vi "GetFileSpace.vi"() -> ()   [LabVIEW 2010]
uses:
  <vilib>/addons/h5labview2/dataset/H5D.lvlib
  <vilib>/addons/h5labview2/dataset/H5Dwrite.llb/H5Dwrite.xnode
  <vilib>/addons/h5labview2/space/H5S.lvlib
  <vilib>/addons/h5labview2/base/H5Equery.vi
  <vilib>/addons/h5labview2/base/lib_path.vi
  <vilib>/addons/h5labview2/base/hid_t.ctl
  fpga-bitfile-ref.ctl
panel:
  in  "Exp_params":T3={"filename"="201612011532", "ExpFilePath"=path "\\\\10.0.0.7\\takada2/DATA/HBT6/data/Test/201612011532.h5", "File Ref list"=[16777216, 33554432], "sweep_dim"=[4, 2], "sweep_list"=[], "readout_list"=["ADC0", "ADC1"], "Sweep instrument bools"=[[0, 0], [0, 0], [0, 0], [0, 0], [0, 0], [0, 0], [0, 0], [0, 0], [0, 0], [0, 0], [0, 0], [0, 0], [0, 0], [0, 0], [0, 0], [0, 0], [0, 0], [0, 0], [0, 0], [0, 0], [0, 0], [0, 0], [0, 0], [0, 0], [0, 0], [0, 0], [0, 0], [0, 0], [0, 0], [0, 0], [0, 0]], "Read out instrument bools"=[[1, 0]], "Experimental bool list"=[FALSE, TRUE], "Initial move"=[{"Name"="None", "kind"=100, "Value"=0.0}], "FPGA Ref"=refnum, "Inst_parameters"={"ConfigFilePath"=path "\\\\10.0.0.7\\takada2/DATA/HBT6/data/Configs/HBT6_ramp_1.h5", "Inst_list"=["ADC", "AWG", "Freq", "Power", "sus", "rus", "rls", "sls", "suq", "suu", "sur", "suc", "sul", "ruq", "ruu", "rur", "ruc", "rul", "rlq", "rlu", "rlr", "rlc", "rll", "slq", "slu", "slr", "slc", "sll", "tu", "t", "tl", "fast_sequence"], "fast_mode"=[1, 1], "Wait_times"=[1, 1, 1, 1], "Inst_array"=[{"Kind"=0, "Strings"=["ADC", "", "V", "ADC0;ADC1", "V;V", "1.0;1.0"], "uint64s"=[10, 2, 250000, 0, 100, 10106, 1000000, 1, 0, 1], "Doubles"=[1.0], "DAQmx take out list"=[]}, {"Kind"=7, "Strings"=["AWG", "10.0.0.4", "", "C:\\Documents and Settings\\Bauerle\\Mes documents\\Bautze\\FPGA-clean_works_1.13.6_batchtest\\Python\\AWG", "dummy", "SAWnstrig_v4.py"], "uint64s"=[2, 0, 0, 3, 0, 0, 0, 0, 0, 0, 0, 0, 0, 0], "Doubles"=[1200000000.0, 1.0, 0.0, 1.0, 0.0, 1.0, 0.0, 1.0, 0.0, 1.0, 0.0, 1.0, 0.0], "DAQmx take out list"=[]}, {"Kind"=6, "Strings"=["Freq", "0:19", "GHz"], "uint64s"=[1, 0, 0, 0, 2, 0, 0, 0], "Doubles"=[2.0, -30.0, 200.0, 100.0, 0.0, 6.000999927520752, 9.000000318337698e-06, 30.0, -145.0], "DAQmx take out list"=[]}, {"Kind"=6, "Strings"=["Power", "0:19", "GHz"], "uint64s"=[1, 0, 1, 0, 2, 0, 0, 0], "Doubles"=[2.0, -30.0, 200.0, 100.0, 0.0, 6.000999927520752, 9.000000318337698e-06, 30.0, -145.0], "DAQmx take out list"=[]}, {"Kind"=4, "Strings"=["sus", "10.0.0.2", "mV"], "uint64s"=[0, 1], "Doubles"=[1.0, -1.0, 1.0, -1.0, 1.0], "DAQmx take out list"=[]}, {"Kind"=4, "Strings"=["rus", "10.0.0.2", "mV"], "uint64s"=[0, 2], "Doubles"=[1.0, -1.0, 1.0, -1.0, 1.0], "DAQmx take out list"=[]}, {"Kind"=4, "Strings"=["rls", "10.0.0.2", "mV"], "uint64s"=[0, 3], "Doubles"=[1.0, -1.0, 1.0, -1.0, 1.0], "DAQmx take out list"=[]}, {"Kind"=4, "Strings"=["sls", "10.0.0.2", "mV"], "uint64s"=[0, 4], "Doubles"=[1.0, -1.0, 1.0, -1.0, 1.0], "DAQmx take out list"=[]}, {"Kind"=4, "Strings"=["suq", "10.0.0.2", "V"], "uint64s"=[0, 5], "Doubles"=[0.30000001192092896, -2.0, 1.0, -1.0, 1.0], "DAQmx take out list"=[]}, {"Kind"=4, "Strings"=["suu", "10.0.0.2", "V"], "uint64s"=[0, 6], "Doubles"=[0.30000001192092896, -2.0, 1.0, -1.0, 1.0], "DAQmx take out list"=[]}, {"Kind"=4, "Strings"=["sur", "10.0.0.2", "V"], "uint64s"=[0, 7], "Doubles"=[0.30000001192092896, -2.0, 1.0, -1.0, 1.0], "DAQmx take out list"=[]}, {"Kind"=4, "Strings"=["suc", "10.0.0.2", "V"], "uint64s"=[1, 0], "Doubles"=[0.30000001192092896, -2.0, 1.0, -1.0, 1.0], "DAQmx take out list"=[]}, {"Kind"=4, "Strings"=["sul", "10.0.0.2", "V"], "uint64s"=[1, 1], "Doubles"=[0.30000001192092896, -2.0, 1.0, -1.0, 1.0], "DAQmx take out list"=[]}, {"Kind"=4, "Strings"=["ruq", "10.0.0.2", "V"], "uint64s"=[1, 2], "Doubles"=[0.30000001192092896, -2.0, 1.0, -1.0, 1.0], "DAQmx take out list"=[]}, {"Kind"=4, "Strings"=["ruu", "10.0.0.2", "V"], "uint64s"=[1, 3], "Doubles"=[0.30000001192092896, -2.0, 1.0, -1.0, 1.0], "DAQmx take out list"=[]}, {"Kind"=4, "Strings"=["rur", "10.0.0.2", "V"], "uint64s"=[1, 5], "Doubles"=[0.30000001192092896, -2.0, 1.0, -1.0, 1.0], "DAQmx take out list"=[]}, {"Kind"=4, "Strings"=["ruc", "10.0.0.2", "V"], "uint64s"=[1, 6], "Doubles"=[0.30000001192092896, -2.0, 1.0, -1.0, 1.0], "DAQmx take out list"=[]}, {"Kind"=4, "Strings"=["rul", "10.0.0.2", "V"], "uint64s"=[1, 7], "Doubles"=[0.30000001192092896, -2.0, 1.0, -1.0, 1.0], "DAQmx take out list"=[]}, {"Kind"=4, "Strings"=["rlq", "10.0.0.2", "V"], "uint64s"=[2, 0], "Doubles"=[0.30000001192092896, -2.0, 1.0, -1.0, 1.0], "DAQmx take out list"=[]}, {"Kind"=4, "Strings"=["rlu", "10.0.0.2", "V"], "uint64s"=[2, 1], "Doubles"=[0.30000001192092896, -2.0, 1.0, -1.0, 1.0], "DAQmx take out list"=[]}, {"Kind"=4, "Strings"=["rlr", "10.0.0.2", "V"], "uint64s"=[2, 2], "Doubles"=[0.30000001192092896, -2.0, 1.0, -1.0, 1.0], "DAQmx take out list"=[]}, {"Kind"=4, "Strings"=["rlc", "10.0.0.2", "V"], "uint64s"=[2, 3], "Doubles"=[0.30000001192092896, -2.0, 1.0, -1.0, 1.0], "DAQmx take out list"=[]}, {"Kind"=4, "Strings"=["rll", "10.0.0.2", "V"], "uint64s"=[2, 4], "Doubles"=[0.30000001192092896, -2.0, 1.0, -1.0, 1.0], "DAQmx take out list"=[]}, {"Kind"=4, "Strings"=["slq", "10.0.0.2", "V"], "uint64s"=[2, 5], "Doubles"=[0.30000001192092896, -2.0, 1.0, -1.0, 1.0], "DAQmx take out list"=[]}, {"Kind"=4, "Strings"=["slu", "10.0.0.2", "V"], "uint64s"=[2, 6], "Doubles"=[0.30000001192092896, -2.0, 1.0, -1.0, 1.0], "DAQmx take out list"=[]}, {"Kind"=4, "Strings"=["slr", "10.0.0.2", "V"], "uint64s"=[2, 7], "Doubles"=[0.30000001192092896, -2.0, 1.0, -1.0, 1.0], "DAQmx take out list"=[]}, {"Kind"=4, "Strings"=["slc", "10.0.0.2", "V"], "uint64s"=[3, 0], "Doubles"=[0.30000001192092896, -2.0, 1.0, -1.0, 1.0], "DAQmx take out list"=[]}, {"Kind"=4, "Strings"=["sll", "10.0.0.2", "V"], "uint64s"=[3, 1], "Doubles"=[0.30000001192092896, -2.0, 1.0, -1.0, 1.0], "DAQmx take out list"=[]}, {"Kind"=4, "Strings"=["tu", "10.0.0.2", "V"], "uint64s"=[3, 2], "Doubles"=[0.30000001192092896, -2.0, 1.0, -1.0, 1.0], "DAQmx take out list"=[]}, {"Kind"=4, "Strings"=["t", "10.0.0.2", "V"], "uint64s"=[3, 3], "Doubles"=[0.30000001192092896, -2.0, 1.0, -1.0, 1.0], "DAQmx take out list"=[]}, {"Kind"=4, "Strings"=["tl", "10.0.0.2", "V"], "uint64s"=[3, 4], "Doubles"=[0.30000001192092896, -2.0, 1.0, -1.0, 1.0], "DAQmx take out list"=[]}, {"Kind"=9, "Strings"=["fast_sequence", "10.0.0.2", "V"], "uint64s"=[6661, 300, 200, 0, 0, 1, 2, 3, 4, 5, 6, 7, 16, 17, 18, 19, 20, 21, 22, 23, 0], "Doubles"=[0.5, -0.5, -1.0, -1.0], "DAQmx take out list"=[]}]}} {"File Ref list" format="%.0x"}
  in  "count":i32
  in  "temp data":dbl[][][](array[numeric])
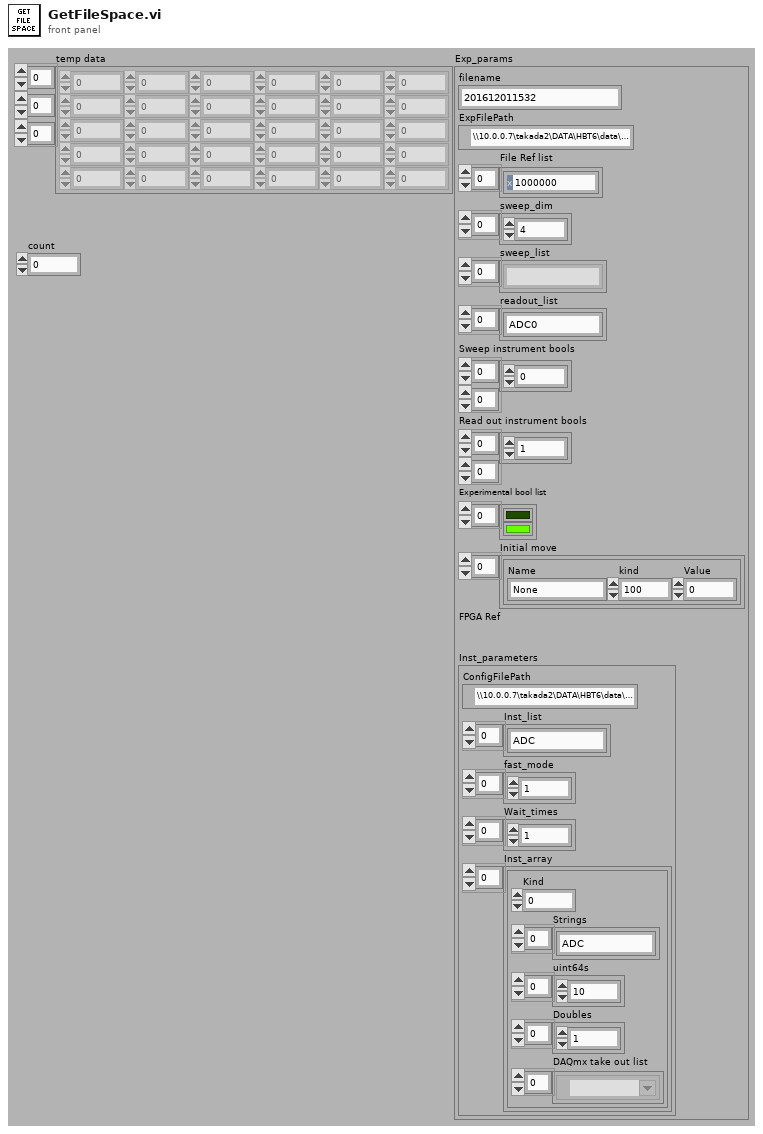
[diagram p1: front panel]
types:
  T1 = typedef "hid_t.ctl" = i32
  T2 = typedef "fpga-bitfile-ref.ctl" = refnum<k20>
  T3 = cluster{"filename":string, "ExpFilePath":path, "File Ref list":T1[], "sweep_dim":u64[], "sweep_list":string[], "readout_list":string[], "Sweep instrument bools":u64[][], "Read out instrument bools":u64[][], "Experimental bool list":bool[], "Initial move":cluster{"Name":string, "kind":u64, "Value":dbl}[], "FPGA Ref":T2, "Inst_parameters":cluster{"ConfigFilePath":path, "Inst_list":string[], "fast_mode":u8[], "Wait_times":u64[], "Inst_array":cluster{"Kind":u16, "Strings":string[], "uint64s":u64[], "Doubles":dbl[], "DAQmx take out list":refnum<k21>[]}[]}}
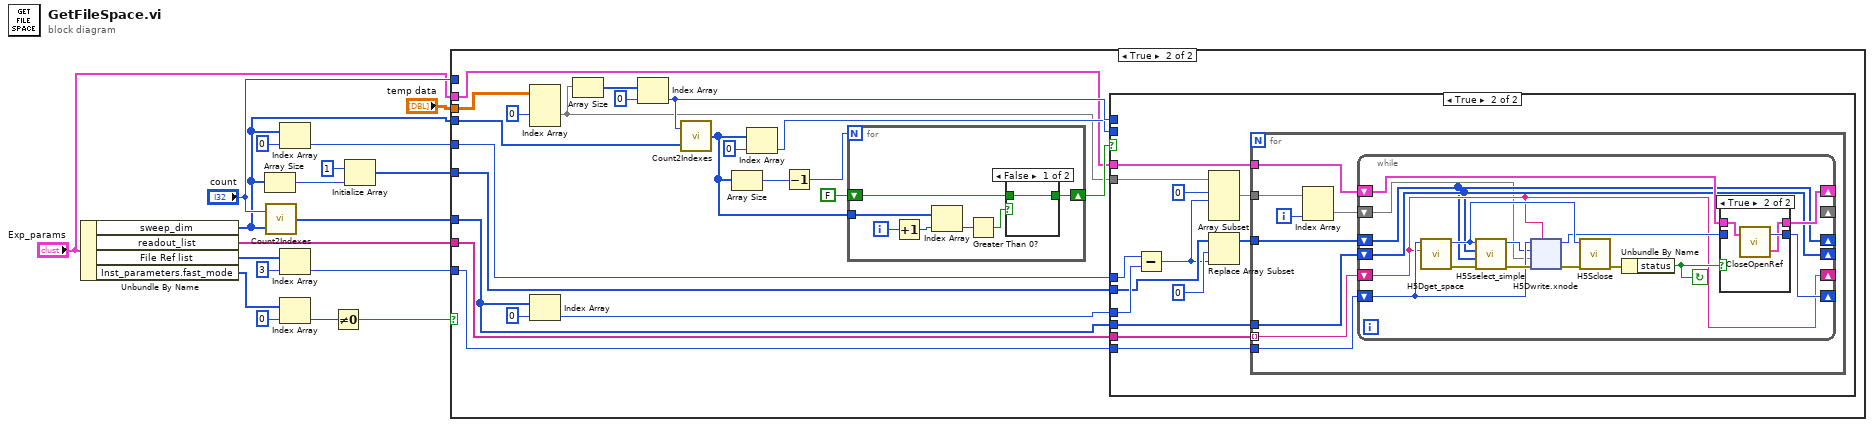
[diagram p0: block diagram]
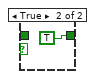
[diagram p5: hidden frame]
diagram:
  n1 = Unbundle By Name("Exp_params") -> ("sweep_dim"=w9:u64[], "readout_list"=w2:string[], "File Ref list"=w4:T1[], "Inst_parameters.fast_mode"=w16:u8[])
  n2 = Array Size(array=w9) -> (size(s)=w8:i32)
  n3 = call "Count2Indexes.vi"("sweep_dim"=w9, "Count"="count") -> ("Indexes"=w12:u64[])
  n4 = Index Array(array=w9, index=0) -> (element=w10:u64)
  n5 = Index Array(array=w4, index=3) -> (element=w3:T1)
  n6 = Index Array(array=w16, index=0) -> (element=w17:u8)
  n7 = Not Equal To 0?(x=w17) -> (x != 0?=w15:bool)
  n8 = Initialize Array(1, w8) -> (w6:i32[])
  n9 = case shown="True" w15 {
    tunnel: "temp data" -> [_ w40]
    tunnel: w9 -> [_ w29]
    tunnel: "count" -> [_ _]
    tunnel: w12 -> [_ w22]
    tunnel: w10 -> [_ w26]
    tunnel: w6 -> [_ w25]
    tunnel: w3 -> [_ w21]
    tunnel: w2 -> [_ w20]
    tunnel: "Exp_params" -> [_ w19]
    frame False {
    }
    frame True {
      n10 = Index Array(array=w40, index (dim 1)=0) -> (element=w24:dbl[][])  [unwired: 2 in]
      n11 = Index Array(array=w22, index=0) -> (element=w27:u64)
      n12 = Array Size(array=w24) -> (size(s)=w23:i32[])
      n13 = Index Array(array=w23, index=0) -> (element=w33:i32)
      n14 = call "Count2Indexes.vi"("sweep_dim"=w29, "Count"=w33) -> ("Indexes"=w31:u64[])
      n15 = Array Size(array=w31) -> (size(s)=w36:i32)
      n16 = Index Array(array=w31, index=0) -> (element=w28:u64)
      n17 = Decrement(x=w36) -> (x-1=w35:i32)
      n18 = for {
        N: w35 -> [_]
        shift-right: [w107] -> w34
        shift-left: FALSE -> [w106]
        tunnel: w31 -> [w104]
        i -> [w105]
        n19 = Increment(x=w105) -> (x+1=w103:i32)
        n20 = Index Array(array=w104, index=w103) -> (element=w101:u64)
        n21 = Greater Than 0?(x=w101) -> (x > 0?=w102:bool)
        n22 = case shown="False" w102 {
          tunnel: [w108 TRUE] -> w107
          tunnel: w106 -> [w108 _]
          frame False {
          }
          frame True {
          }
        }
      }
      n23 = case shown="True" w34 {
        tunnel: w33 -> [_ _]
        tunnel: w28 -> [_ _]
        tunnel: w27 -> [_ w52]
        tunnel: w26 -> [_ w53]
        tunnel: w25 -> [_ w51]
        tunnel: w24 -> [_ w44]
        tunnel: w22 -> [_ w49]
        tunnel: w21 -> [_ w47]
        tunnel: w20 -> [_ w46]
        tunnel: w19 -> [_ w45]
        frame False {
        }
        frame True {
          n24 = Subtract(x=w53, y=w52) -> (x-y=w42:u64)
          n25 = Array Subset(array=w44, index (row)=0, length (row)=w42) -> (w41:dbl[][])  [unwired: 2 in]
          n26 = Replace Array Subset(array=w51, new element=w42, index=0) -> (w48:i32[])
          n27 = for {
            tunnel: w49 -> [w61]
            tunnel: w48 -> [w60]
            tunnel: w47 -> [w59]
            tunnel: w46 -> [w58] mode=indexing
            tunnel: w45 -> [w57]
            tunnel: w41 -> [w56]
            i -> [w55]
            n28 = Index Array(array=w56, index (col)=w55) -> (element=w54:dbl[])  [unwired: 1 in]
            n29 = while {
              shift-right: [w69] -> _
              shift-left: w59 -> [w75]
              shift-right: [w67] -> _
              shift-left: w57 -> [w68]
              shift-right: _ -> [_]
              shift-left: w54 -> [w62]
              shift-right: [w64] -> _
              shift-left: w61 -> [w64]
              shift-right: [w63] -> _
              shift-left: w60 -> [w63]
              shift-right: [w65] -> _
              shift-left: w58 -> [w65]
              stop <- w66 continue-if-true
              n30 = call <vilib>:"H5Dget_space.vi"("obj (.)"=w65, "ref in"=w75) -> ("error out"=w77:errorcluster, "space out"=w73:T1)  [unwired: 8 in]
              n31 = call <vilib>:"H5Sselect_simple.vi"("error in (no error)"=w77, "count"=w63, "start"=w64, "space in"=w73) -> ("error out"=w76:errorcluster, "space out"=w74:T1)  [unwired: 6 in]
              n32 = xnode "H5Dwrite.xnode"("dataset name"=w65, "error in (no error)"=w76, "data"=w62, "file space"=w74, "ref in"=w75) -> ("error out"=w72:errorcluster, "ref out"=w70:i32)  [unwired: 2 in, 1 out]
              n33 = call <vilib>:"H5Sclose.vi"("error in (no error)"=w72, "space in"=w73) -> ("error out"=w71:errorcluster)  [unwired: 9 in]
              n34 = Unbundle By Name(w71) -> ("status"=w66:bool)
              n35 = case shown="True" w66 {
                tunnel: w70 -> [w79 _]
                tunnel: [w79 w81] -> w69
                tunnel: w68 -> [w78 w82]
                tunnel: [w78 w80] -> w67
                frame False {
                }
                frame True {
                  n36 = call "CloseOpenRef.vi"("Exp_params"=w82) -> ("Exp_params_out"=w80:T3, "group out"=w81:T1)  [unwired: 1 in]
                }
              }
            }
          }
        }
      }
    }
  }
